vi "Handle.vi"(11 "Hello World Event in":refnum<class "Hello World Event.lvclass">) -> (2 "Destroy?":bool, 3 "Hello World Event out":refnum<class "Hello World Event.lvclass">)   [LabVIEW 2021, in "Hello World Event.lvlib" / "Hello World Event.lvclass"]
uses:
  Hello World Event.lvclass
  Hello World Event.lvclass/Hello World Event.ctl
  jettl/jettl/Event jettl/Event jettl.lvclass
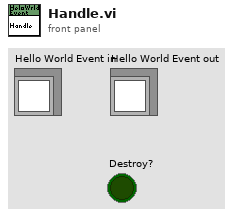
[diagram p1: front panel]
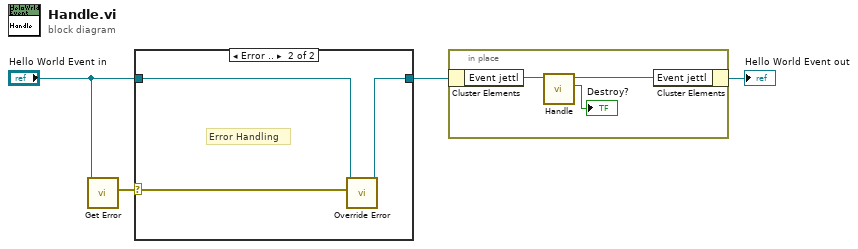
[diagram p0: block diagram]
diagram:
  n1 = call-dynamic "Get Error.vi"("Hello World Event in"="Hello World Event in") -> ("Error"=w3:errorcluster)  [unwired: 10 in]
  n2 = case shown="Error .." w3 {
    selector: w3 -> [_ w6]
    tunnel: "Hello World Event in" -> [w5 w8]
    tunnel: [w5 w7] -> w2
    frame No Error {
    }
    frame Error {
      # "Error Handling"
      n3 = call-dynamic "Override Error.vi"("Error"=w6, "Hello World Event in"=w8) -> ("Hello World Event out"=w7:refnum<class "Hello World Event.lvclass">)  [unwired: 9 in]
    }
  }
  n4 = in-place {
    n5 = in-place-cluster #1(w2) -> ("Event jettl"=w10:refnum<class "Event jettl.lvclass">)
    n6 = call-dynamic "Handle.vi"("jettl in"=w10) -> ("Destroy?"=→"Destroy?":bool, "jettl out"=w9:refnum<class "Event jettl.lvclass">)  [unwired: 9 in]
    n7 = in-place-cluster #1("Event jettl"=w9) -> (→"Hello World Event out":refnum<class "Hello World Event.lvclass">)
  }
